vi "运维调试_五参数.vi"(11 "编号":string="001") -> ()   [LabVIEW 2016, in "斯坦道多参数.lvlib"]
uses:
  <vilib>/Utility/miscctls.llb/LVPointTypeDef.ctl
  <vilib>/Plasmionique/MB Master/MB_Master/MB_Master.lvclass
  <vilib>/Utility/config.llb/NI_LVConfig.lvlib
panel:
  out "权限等级":string
  in  "ORP校准":bool
  in  "ORP探头选择":u16(ring) items=["YL型", "MQ型", "NAQ型"]
  in  "ORP启用":bool
  in  "水样测量时间":dbl caption="水样测量时间:"
  in  "自动断线重连":bool=TRUE
  in  "打开modbus":bool
  out "选项卡控件":enum32{"选项卡 1", "选项卡 2"}(tab)
  in  "VISA资源名称":refnum<visa-resource-name> caption="串口"
  in  "IP":string="localhost" caption="IP:"
  in  "Port":u16=502 caption="Port:"
  in  "连接方式":u16(ring) items=["Modbus RTU", "Modbus TCP"]
  in  "藻密度校准":bool
  in  "密码锁":bool
  in  "藻密度探头选择":u16(ring) items=["YL型", "MQ型", "NAQ型"]
  in  "叶绿素a探头选择":u16(ring) items=["YL型", "MQ型", "NAQ型"]
  in  "浊度探头选择":u16(ring) items=["YL型", "MQ型", "NAQ型"]
  in  "电导率探头选择":u16(ring) items=["YL型", "MQ型", "NAQ型"]
  in  "DO探头选择":u16(ring) items=["YL型", "MQ型", "NAQ型"]
  in  "pH探头选择":u16(ring) items=["YL型", "MQ型", "NAQ型"]
  in  "设置页返回":bool
  in  "藻密度":bool
  in  "叶绿素a启用":bool
  in  "Temp":bool
  in  "Cond":bool
  in  "Turb":bool
  in  "DO":bool
  in  "pH":bool
  in  "周期设置":bool
  out "当前串口":string
  out "运行状态":u16(ring) items=["空闲", "水样测试", "标样核查"]
  in  "叶绿素a校准":bool
  in  "停止":bool
  in  "标样核查":bool
  in  "水样测试":bool
  in  "设置":bool
  in  "水温校准":bool
  in  "浊度校准":bool
  in  "溶解氧校准":bool
  in  "电导率校准":bool
  in  "pH校准":bool
  in  "探头校正返回":bool
  in  "探头校正":bool
  out "检测值":T1(array[cluster])
  # "请设置仪器连接方式"
  # "请选择要启用的参数"
  # "min"
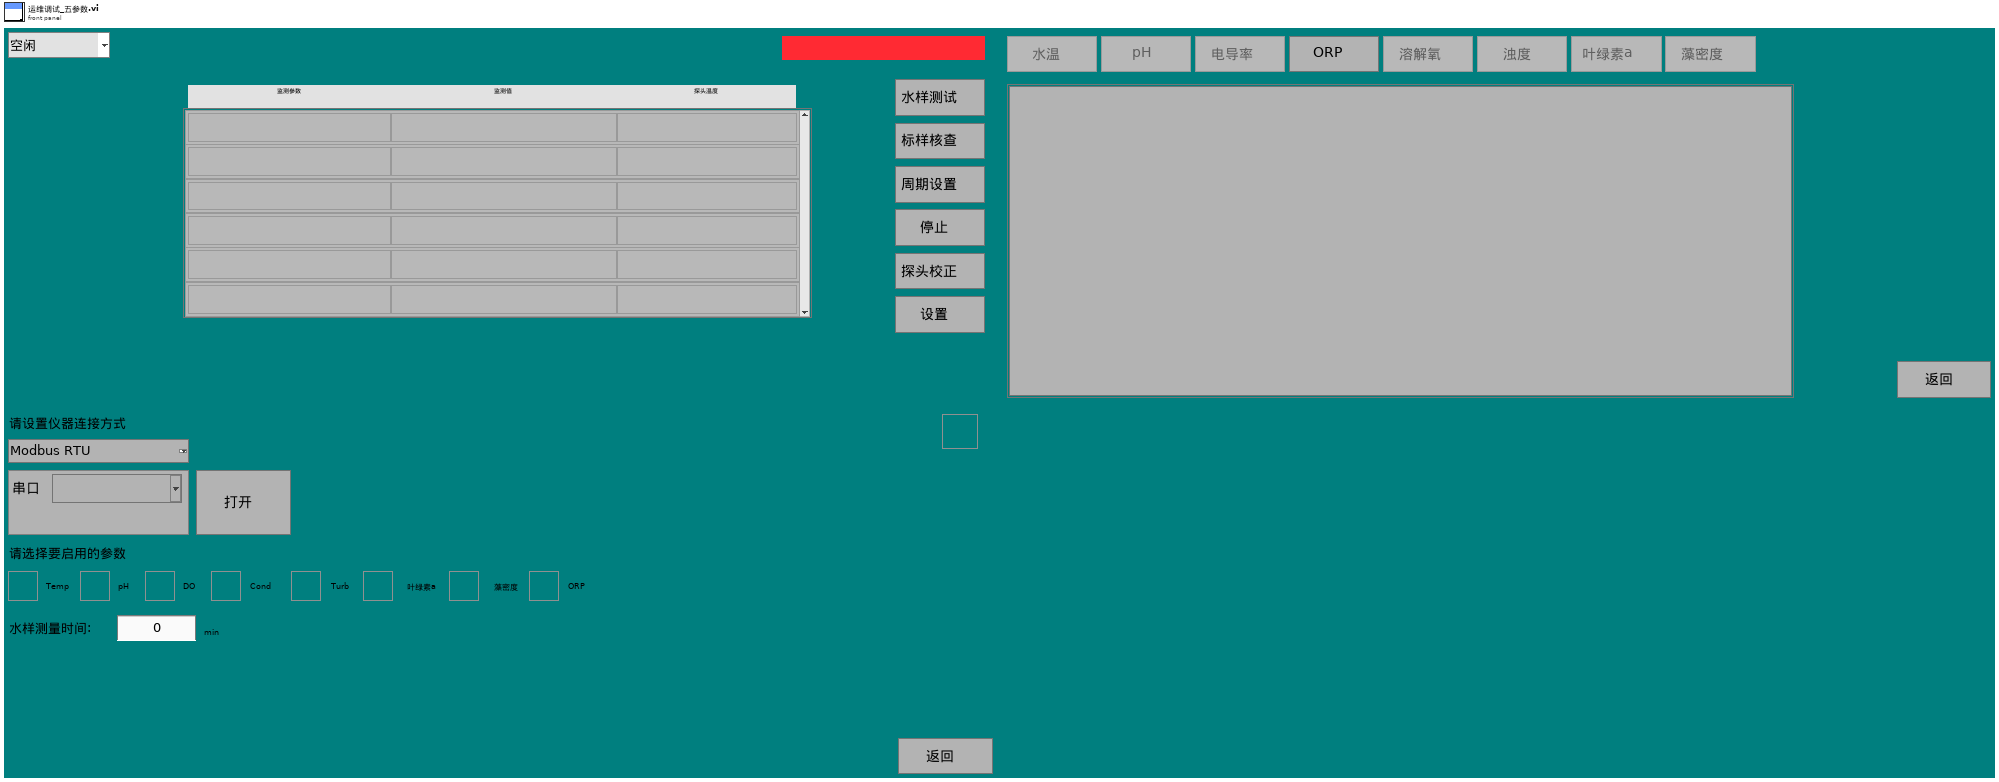
[diagram p1: front panel]
types:
  T1 = cluster{"监测参数1":string, "浓度1":string, "探头温度1":string}[]
  T2 = typedef "LVPointTypeDef.ctl" = cluster{"Horizontal":i16, "Vertical":i16}
  T3 = enum8{"Enabled", "Disabled", "Disabled and Grayed Out"}
  T4 = cluster{"pH探头选择":u16, "DO探头选择":u16, "电导率探头选择":u16, "浊度探头选择":u16, "叶绿素a探头选择":u16, "蓝绿藻探头选择":u16, "orp探头选择":u16}
  T5 = cluster{"温度测量值":sgl, "DO%":sgl, "DOmg/L":sgl, "温度偏移修正值":sgl}
  T6 = cluster{"周期设置类型":enum16{"定点启动", "间隔启动"}, "定时功能启用":bool, "定时间隔":u32, "24H周期设置":bool[]}
  T7 = enum32{"Bad", "Idle", "Run top level", "Running"}
  T8 = typedef "LVDateTimeRec.ctl" = cluster{"秒数的小数部分":dbl, "秒":i32, "分":i32, "时":i32, "日":i32, "月":i32, "年":i32, "天数（周）":i32, "天数（年）":i32, "DST":i32}
  T9 = typedef "NI_LVConfig.lvlib/Config Data RefNum.ctl" = refnum<k1>
  T10 = cluster{"pH校准VI引用句柄":refnum<vi>, "DO校准VI引用句柄":refnum<vi>, "COND校准VI引用句柄":refnum<vi>, "TURB校准VI引用句柄":refnum<vi>, "CHLA校准VI引用句柄":refnum<vi>, "BGA校准VI引用句柄":refnum<vi>, "ORP校准VI引用句柄":refnum<vi>}
  T11 = cluster{"数据保存间隔":dbl, "水温标样值":dbl, "pH标样值":dbl, "溶解氧标样值":dbl, "电导率标样值":dbl, "浊度标样值":dbl}
  T12 = cluster{"baud rate (bps)":u32, "stop bits":u16, "parity":u16, "flow control":u16, "timeout":u32, "retries":i32}
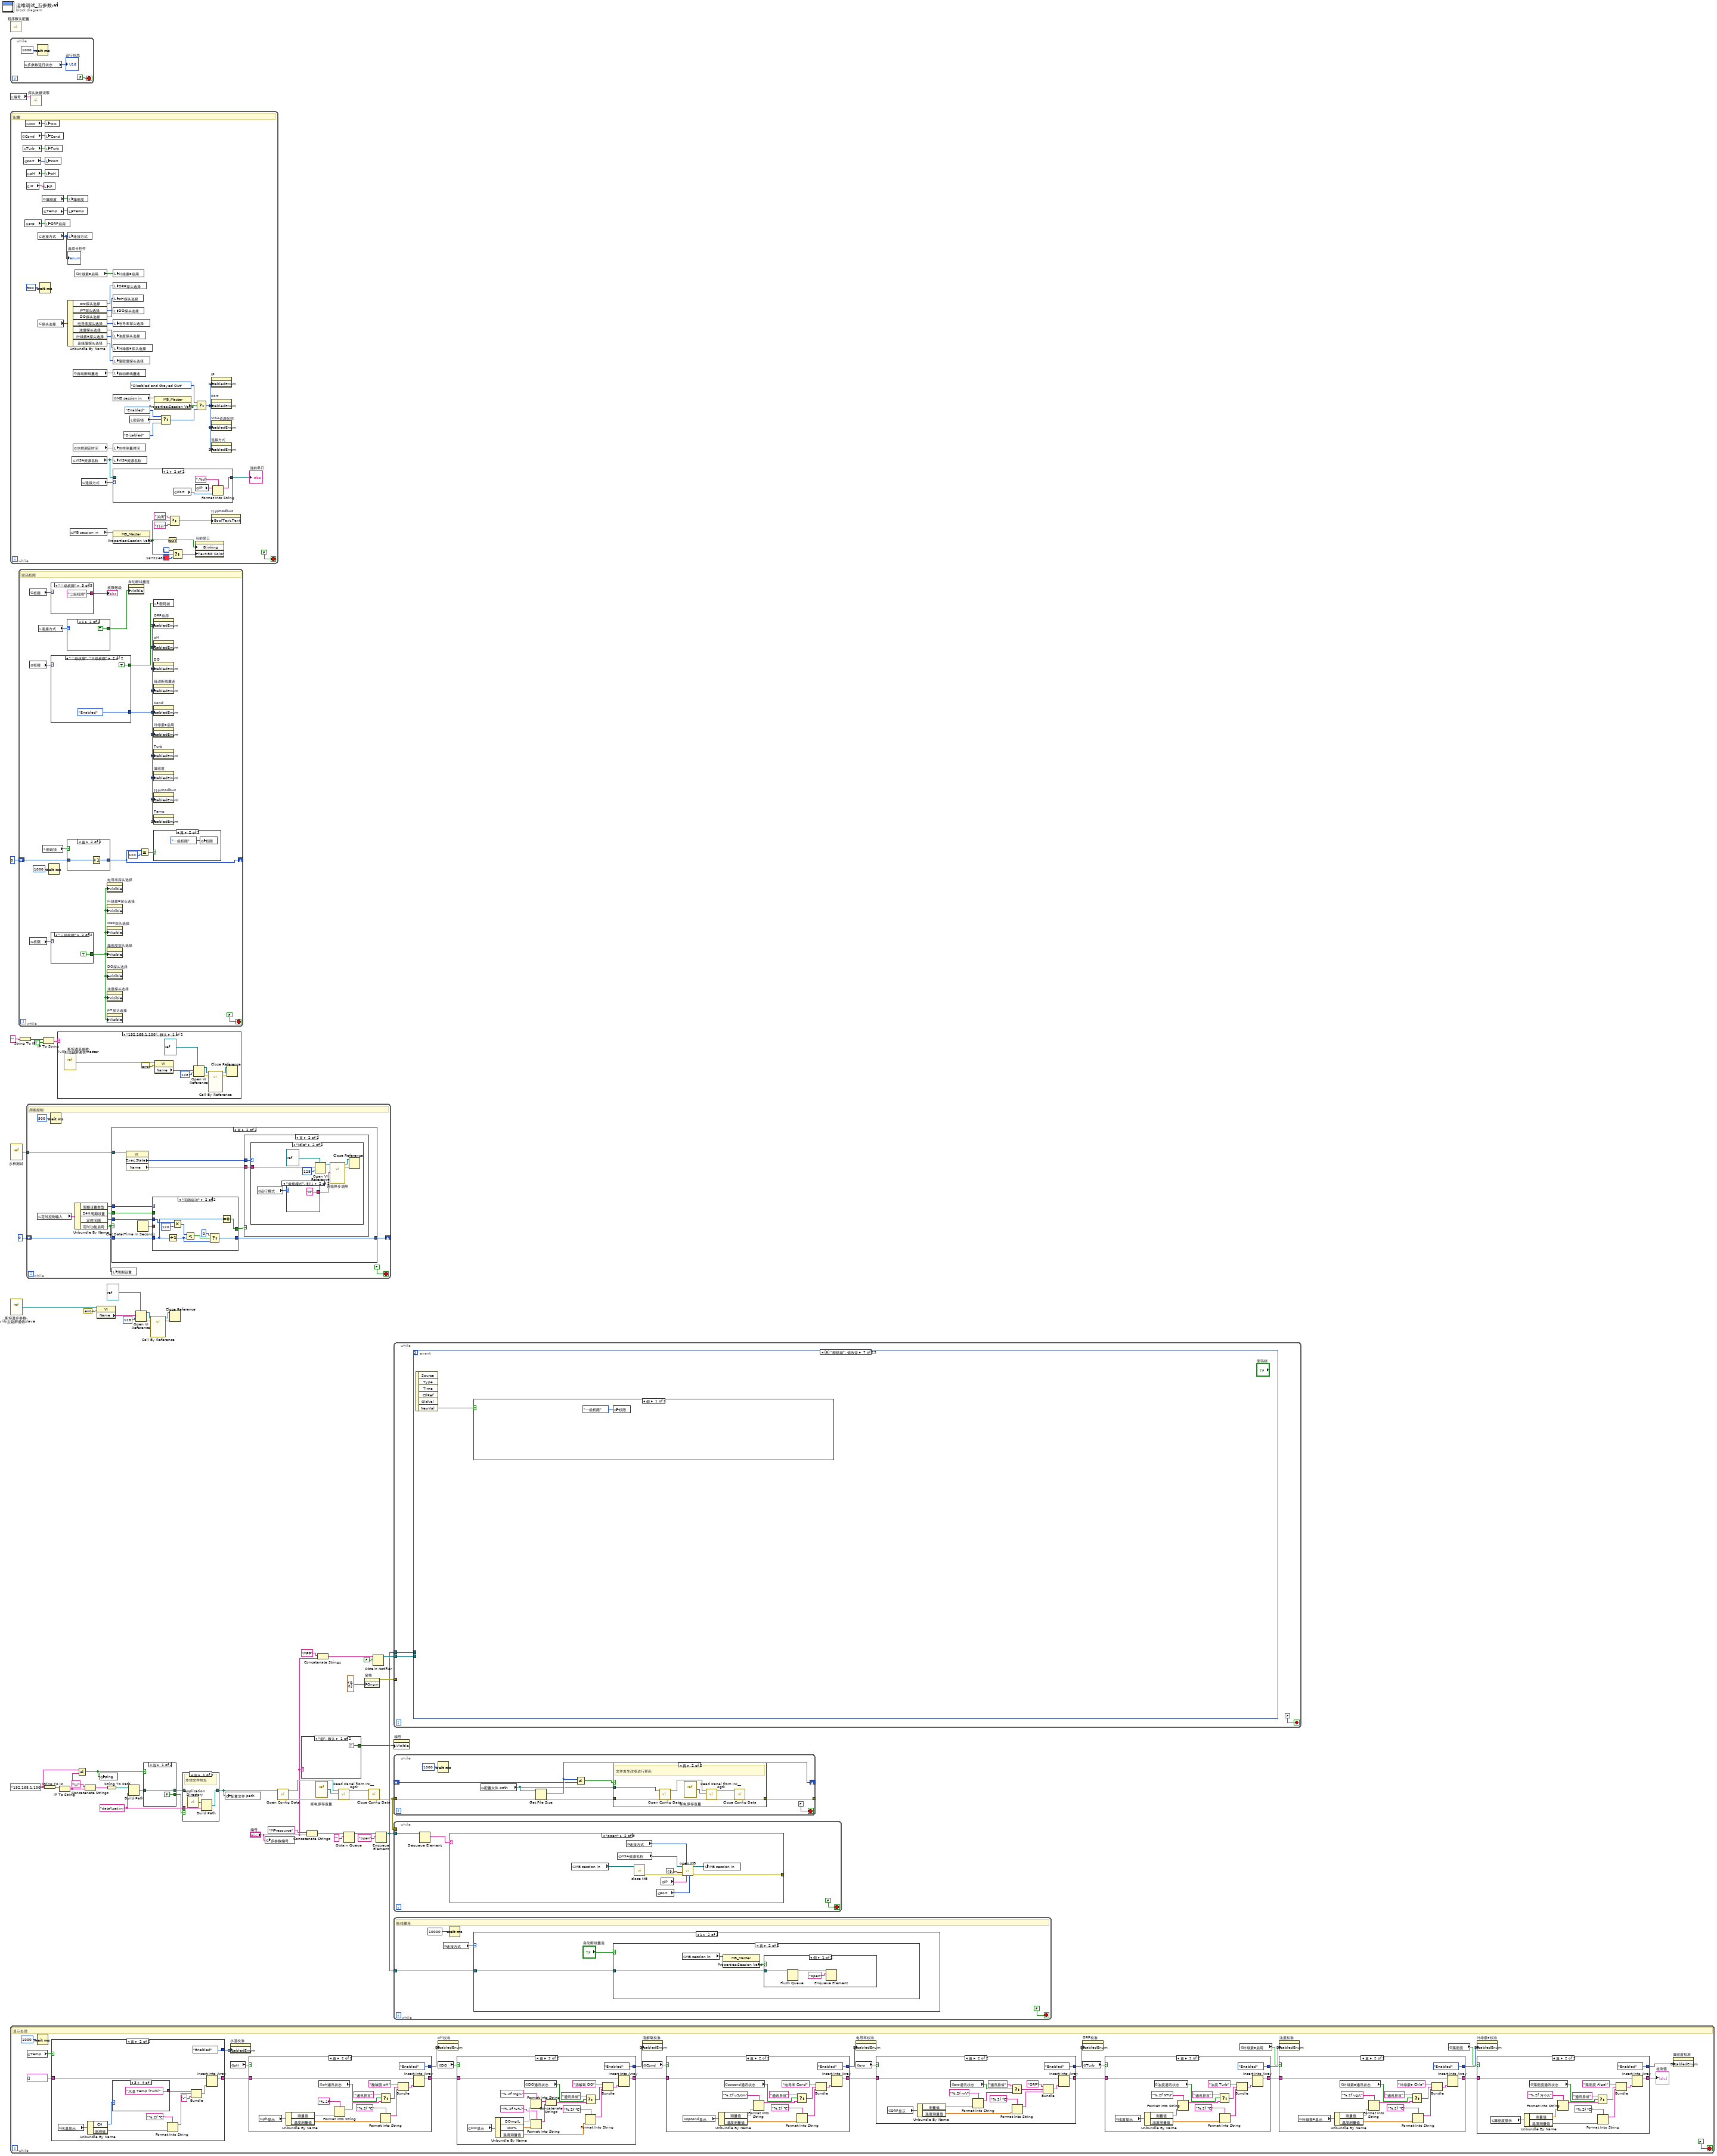
[diagram p0: block diagram]
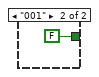
[diagram p2: hidden frame]
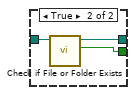
[diagram p4: hidden frame]
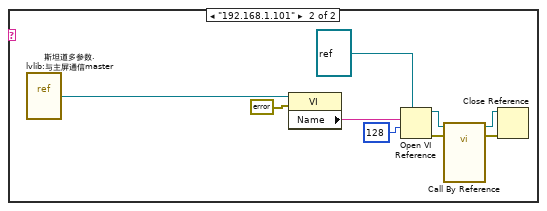
[diagram p6: hidden frame]
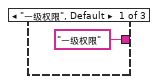
[diagram p13: hidden frame]
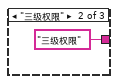
[diagram p14: hidden frame]
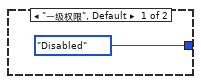
[diagram p15: hidden frame]
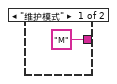
[diagram p20: hidden frame]
diagram:
  w16 = "data\\set.ini" ("名称或相对路径")
  w8 = "192.168.1.100" ("名称")
  n1 = call "程序默认配置.vi"() -> ()  [unwired: 11 in, 1 out]
  n2 = while {
    stop <- FALSE stop-if-true
    n3 = global read "多参数全局变量.vi" "多参数运行状态"() -> (→"运行状态":u16)
    n4 = Wait (ms)(milliseconds to wait=u32 1000 ("等待时间（毫秒）")) -> ()  [unwired: 1 out]
  }
  n5 = local read "编号"() -> (w3:string)
  n6 = while {
    stop <- FALSE stop-if-true
    # "配置"
    n7 = global read "断电保存变量.vi" "Cond"() -> (w91:bool)
    n8 = global read "断电保存变量.vi" "Turb"() -> (w90:bool)
    n9 = global read "断电保存变量.vi" "Port"() -> (w69:u16)
    n10 = global read "断电保存变量.vi" "orp"() -> (w54:bool)
    n11 = global read "断电保存变量.vi" "DO"() -> (w92:bool)
    n12 = global read "断电保存变量.vi" "pH"() -> (w93:bool)
    n13 = global read "断电保存变量.vi" "IP"() -> (w70:string)
    n14 = global read "断电保存变量.vi" "连接方式"() -> (w62:u16)
    "选项卡控件" <- w62
    n15 = global read "断电保存变量.vi" "探头选择"() -> (w80:T4)
    n16 = Wait (ms)(milliseconds to wait=u32 500 ("等待时间（毫秒）")) -> ()  [unwired: 1 out]
    n17 = global read "断电保存变量.vi" "藻密度"() -> (w88:bool)
    n18 = global read "断电保存变量.vi" "Temp"() -> (w94:bool)
    n19 = local write "IP"(w70) -> ()
    n20 = local write "DO"(w92) -> ()
    n21 = local write "Cond"(w91) -> ()
    n22 = local write "Turb"(w90) -> ()
    n23 = local write "Port"(w69) -> ()
    n24 = local write "pH"(w93) -> ()
    n25 = local write "ORP启用"(w54) -> ()
    n26 = local write "藻密度"(w88) -> ()
    n27 = local write "Temp"(w94) -> ()
    n28 = local write "连接方式"(w62) -> ()
    n29 = Unbundle By Name(w80) -> ("orp探头选择"=w53:u16, "pH探头选择"=w63:u16, "DO探头选择"=w79:u16, "电导率探头选择"=w78:u16, "浊度探头选择"=w77:u16, "叶绿素a探头选择"=w76:u16, "蓝绿藻探头选择"=w75:u16)
    n30 = global read "多参数全局变量.vi" "MB session in"() -> (w84:refnum<class "MB_Master.lvclass">)
    n31 = global read "断电保存变量.vi" "VISA资源名称"() -> (w66:refnum<visa-resource-name>)
    n32 = global read "断电保存变量.vi" "自动断线重连"() -> (w57:bool)
    n33 = global read "断电保存变量.vi" "水样测定时间"() -> (w56:dbl)
    n34 = global read "断电保存变量.vi" "叶绿素a启用"() -> (w89:bool)
    n35 = global read "断电保存变量.vi" "连接方式"() -> (w67:u16)
    n36 = local write "叶绿素a启用"(w89) -> ()
    n37 = local write "ORP探头选择"(w53) -> ()
    n38 = local write "pH探头选择"(w63) -> ()
    n39 = local write "DO探头选择"(w79) -> ()
    n40 = local write "电导率探头选择"(w78) -> ()
    n41 = local write "浊度探头选择"(w77) -> ()
    n42 = local write "叶绿素a探头选择"(w76) -> ()
    n43 = local write "藻密度探头选择"(w75) -> ()
    n44 = local write "自动断线重连"(w57) -> ()
    n45 = global read "多参数全局变量.vi" "MB session in"() -> (w87:refnum<class "MB_Master.lvclass">)
    n46 = local write "水样测量时间"(w56) -> ()
    n47 = local write "VISA资源名称"(w66) -> ()
    n48 = case shown="1" w67 {
      tunnel: w66 -> [w96 _]
      tunnel: [w96 w97] -> w65
      frame 0, Default {
      }
      frame 1 {
        n49 = global read "断电保存变量.vi" "Port"() -> (w98:u16)
        n50 = global read "断电保存变量.vi" "IP"() -> (w100:string)
        n51 = Format Into String(format string=":%d" ("格式字符串"), initial string=w100, w98) -> (resulting string=w97:string)  [unwired: 1 in, 1 out]
      }
    }
    "当前串口" <- w65
    n52 = property class="MB_Master"(reference=w84) -> ("Properties:Session Valid"=w61:bool)  [unwired: 1 in, 2 out]
    n53 = local read "密码锁"() -> (w74:bool)
    n54 = property class="MB_Master"(reference=w87) -> ("Properties:Session Valid"=w86:bool)  [unwired: 1 in, 2 out]
    n55 = Select(t=T3."Enabled" ("f"), s=w74, f=T3."Disabled") -> (s? t:f=w72:T3)
    n56 = Not(x=w61) -> (.not. x?=w64:bool)
    n57 = Select(t="关闭" ("布尔文本.文本"), s=w61, f="打开" ("布尔文本.文本")) -> (s? t:f=w81:string)
    n58 = Select(t=u32 16777216, s=w61, f=u32 16722483) -> (s? t:f=w58:u32)
    n59 = property on="当前串口" class="Str"("Blinking"=w64, "Text.BG Color"=w58) -> ()  [unwired: 2 in, 2 out]
    n60 = Select(t=T3."Disabled and Grayed Out" ("禁用"), s=w86, f=w72) -> (s? t:f=w68:T3)
    n61 = property on="IP" class="Str"("DisabledEnum"=w68) -> ()  [unwired: 2 in, 2 out]
    n62 = property on="Port" class="DigNum (严格)"("DisabledEnum"=w68) -> ()  [unwired: 2 in, 2 out]
    n63 = property on="VISA资源名称" class="VISAName"("DisabledEnum"=w68) -> ()  [unwired: 2 in, 2 out]
    n64 = property on="连接方式" class="Ring (严格)"("DisabledEnum"=w68) -> ()  [unwired: 2 in, 2 out]
    n65 = property on="打开modbus" class="Bool"("BoolText.Text"=w81) -> ()  [unwired: 2 in, 2 out]
  }
  n66 = vi-ref "水样测试.vi"() -> (w39:refnum<vi>)
  n67 = vi-ref "斯坦道多参数.lvlib:主副屏通信slave.vi"() -> (w21:refnum<vi>)
  n68 = while {
    stop <- FALSE stop-if-true
    # "显示处理"
    n69 = global read "断电保存变量.vi" "Temp"() -> (w125:bool)
    n70 = Wait (ms)(milliseconds to wait=u32 1000 ("等待时间（毫秒）")) -> ()  [unwired: 1 out]
    n71 = case shown="真" w125 {
      tunnel: [w252 w257] -> w122
      tunnel: T1 [] ("数组") -> [w252 w258]
      tunnel: [T3."Disabled and Grayed Out" ("禁用") T3."Enabled" ("禁用")] -> w109
      frame False {
      }
      frame True {
        n72 = global read "多参数全局变量.vi" "水温显示"() -> (w255:cluster{"CH":u16, "监测值":dbl, "温度偏移修正值":sgl})
        n73 = Unbundle By Name(w255) -> ("CH"=w254:u16, "监测值"=w253:dbl)
        n74 = case shown="3" w254 {
          tunnel: ["水温 Temp (pH)" ("监测参数1") "水温 Temp (Cond)" ("监测参数1") "水温 Temp (DO)" ("监测参数1") "水温 Temp (Turb)" ("监测参数1")] -> w262
          frame 0, Default {
          }
          frame 1 {
          }
          frame 2 {
          }
          frame 3 {
          }
        }
        n75 = Format Into String(format string="%.2f ℃" ("格式字符串"), w253) -> (resulting string=w261:string)  [unwired: 2 in, 1 out]
        n76 = Bundle("监测参数1"=w262, w261, "探头温度1"="-") -> (w259:cluster{"监测参数1":string, string, "探头温度1":string})  [unwired: 1 in]
        n77 = Insert Into Array(array=w258, new element=w259) -> (w257:T1)  [unwired: 1 in]
      }
    }
    n78 = property on="水温校准" class="Bool"("DisabledEnum"=w109) -> ()  [unwired: 2 in, 2 out]
    n79 = global read "断电保存变量.vi" "pH"() -> (w123:bool)
    n80 = case shown="真" w123 {
      tunnel: [w235 w242] -> w120
      tunnel: w122 -> [w235 w244]
      tunnel: [T3."Disabled and Grayed Out" ("禁用") T3."Enabled" ("禁用")] -> w114
      frame False {
      }
      frame True {
        n81 = global read "多参数全局变量.vi" "ph显示"() -> (w240:cluster{"温度测量值":sgl, "测量值":sgl, "温度偏移修正值":sgl})
        n82 = Unbundle By Name(w240) -> ("测量值"=w250:sgl, "温度测量值"=w248:sgl)
        n83 = global read "多参数全局变量.vi" "ph通讯状态"() -> (w238:bool)
        n84 = Format Into String(format string="%.2f" ("格式字符串"), w250) -> (resulting string=w237:string)  [unwired: 2 in, 1 out]
        n85 = Select(t="通讯异常" ("格式字符串"), s=w238, f=w237) -> (s? t:f=w236:string)
        n86 = Format Into String(format string="%.2f ℃" ("格式字符串"), w248) -> (resulting string=w246:string)  [unwired: 2 in, 1 out]
        n87 = Bundle("监测参数2"="酸碱度 pH", "格式字符串"=w236, w246) -> (w243:cluster{"监测参数2":string, "格式字符串":string, string})  [unwired: 1 in]
        n88 = Insert Into Array(array=w244, new element=w243) -> (w242:T1)  [unwired: 1 in]
      }
    }
    n89 = property on="pH校准" class="Bool"("DisabledEnum"=w114) -> ()  [unwired: 2 in, 2 out]
    n90 = global read "断电保存变量.vi" "DO"() -> (w121:bool)
    n91 = case shown="真" w121 {
      tunnel: [w214 w221] -> w117
      tunnel: w120 -> [w214 w222]
      tunnel: [T3."Disabled and Grayed Out" ("禁用") T3."Enabled" ("禁用")] -> w113
      frame False {
      }
      frame True {
        n92 = global read "多参数全局变量.vi" "DO显示"() -> (w219:T5)
        n93 = Unbundle By Name(w219) -> ("DOmg/L"=w230:sgl, "DO%"=w228:sgl, "温度测量值"=w232:sgl)
        n94 = global read "多参数全局变量.vi" "DO通讯状态"() -> (w217:bool)
        n95 = Format Into String(format string="%.2f mg/L" ("格式字符串"), w230) -> (resulting string=w227:string)  [unwired: 2 in, 1 out]
        n96 = Format Into String(format string="(%.2f %%)" ("格式字符串"), w228) -> (resulting string=w226:string)  [unwired: 2 in, 1 out]
        n97 = Concatenate Strings(w227, w226) -> (w216:string)
        n98 = Select(t="通讯异常" ("格式字符串"), s=w217, f=w216) -> (s? t:f=w215:string)
        n99 = Format Into String(format string="%.2f ℃" ("格式字符串"), w232) -> (resulting string=w224:string)  [unwired: 2 in, 1 out]
        n100 = Bundle("监测参数2"="溶解氧 DO", "格式字符串"=w215, w224) -> (w223:cluster{"监测参数2":string, "格式字符串":string, string})  [unwired: 1 in]
        n101 = Insert Into Array(array=w222, new element=w223) -> (w221:T1)  [unwired: 1 in]
      }
    }
    n102 = property on="溶解氧校准" class="Bool"("DisabledEnum"=w113) -> ()  [unwired: 2 in, 2 out]
    n103 = global read "断电保存变量.vi" "Cond"() -> (w119:bool)
    n104 = case shown="真" w119 {
      tunnel: w117 -> [w197 w208]
      tunnel: [w197 w198] -> w102
      tunnel: [T3."Disabled and Grayed Out" ("禁用") T3."Enabled" ("禁用")] -> w112
      frame False {
      }
      frame True {
        n105 = global read "多参数全局变量.vi" "spcond显示"() -> (w205:cluster{"温度测量值":sgl, "测量值":sgl, "温度偏移修正值":sgl})
        n106 = Unbundle By Name(w205) -> ("测量值"=w204:sgl, "温度测量值"=w203:sgl)
        n107 = global read "多参数全局变量.vi" "spcond通讯状态"() -> (w201:bool)
        n108 = Format Into String(format string="%.2f uS/cm" ("格式字符串"), w204) -> (resulting string=w200:string)  [unwired: 2 in, 1 out]
        n109 = Select(t="通讯异常" ("格式字符串"), s=w201, f=w200) -> (s? t:f=w199:string)
        n110 = Format Into String(format string="%.2f ℃" ("格式字符串"), w203) -> (resulting string=w209:string)  [unwired: 2 in, 1 out]
        n111 = Bundle("监测参数2"="电导率 Cond", "格式字符串"=w199, w209) -> (w207:cluster{"监测参数2":string, "格式字符串":string, string})  [unwired: 1 in]
        n112 = Insert Into Array(array=w208, new element=w207) -> (w198:T1)  [unwired: 1 in]
      }
    }
    n113 = property on="电导率校准" class="Bool"("DisabledEnum"=w112) -> ()  [unwired: 2 in, 2 out]
    n114 = global read "断电保存变量.vi" "orp"() -> (w104:bool)
    n115 = case shown="真" w104 {
      tunnel: w102 -> [w129 w140]
      tunnel: [w129 w138] -> w103
      tunnel: [T3."Disabled and Grayed Out" ("禁用") T3."Enabled" ("禁用")] -> w101
      frame False {
      }
      frame True {
        n116 = global read "多参数全局变量.vi" "ORP显示"() -> (w136:cluster{"温度测量值":sgl, "测量值":sgl, "温度偏移修正值":sgl})
        n117 = Unbundle By Name(w136) -> ("测量值"=w135:sgl, "温度测量值"=w134:sgl)
        n118 = global read "多参数全局变量.vi" "orp通讯状态"() -> (w132:bool)
        n119 = Format Into String(format string="%.2f mV" ("格式字符串"), w135) -> (resulting string=w131:string)  [unwired: 2 in, 1 out]
        n120 = Select(t="通讯异常" ("格式字符串"), s=w132, f=w131) -> (s? t:f=w130:string)
        n121 = Format Into String(format string="%.2f ℃" ("格式字符串"), w134) -> (resulting string=w141:string)  [unwired: 2 in, 1 out]
        n122 = Bundle("监测参数2"="ORP", "格式字符串"=w130, w141) -> (w139:cluster{"监测参数2":string, "格式字符串":string, string})  [unwired: 1 in]
        n123 = Insert Into Array(array=w140, new element=w139) -> (w138:T1)  [unwired: 1 in]
      }
    }
    n124 = property on="ORP校准" class="Bool"("DisabledEnum"=w101) -> ()  [unwired: 2 in, 2 out]
    n125 = global read "断电保存变量.vi" "Turb"() -> (w118:bool)
    n126 = case shown="真" w118 {
      tunnel: w103 -> [w180 w191]
      tunnel: [w180 w189] -> w116
      tunnel: [T3."Disabled and Grayed Out" ("禁用") T3."Enabled" ("禁用")] -> w111
      frame False {
      }
      frame True {
        n127 = global read "多参数全局变量.vi" "浊度显示"() -> (w187:cluster{"温度测量值":sgl, "测量值":sgl, "温度偏移修正值":sgl})
        n128 = Unbundle By Name(w187) -> ("测量值"=w186:sgl, "温度测量值"=w185:sgl)
        n129 = global read "多参数全局变量.vi" "浊度通讯状态"() -> (w183:bool)
        n130 = Format Into String(format string="%.2f NTU" ("格式字符串"), w186) -> (resulting string=w182:string)  [unwired: 2 in, 1 out]
        n131 = Select(t="通讯异常" ("格式字符串"), s=w183, f=w182) -> (s? t:f=w181:string)
        n132 = Format Into String(format string="%.2f ℃" ("格式字符串"), w185) -> (resulting string=w193:string)  [unwired: 2 in, 1 out]
        n133 = Bundle("监测参数2"="浊度 Turb", "格式字符串"=w181, w193) -> (w190:cluster{"监测参数2":string, "格式字符串":string, string})  [unwired: 1 in]
        n134 = Insert Into Array(array=w191, new element=w190) -> (w189:T1)  [unwired: 1 in]
      }
    }
    n135 = global read "断电保存变量.vi" "叶绿素a启用"() -> (w115:bool)
    n136 = property on="浊度校准" class="Bool"("DisabledEnum"=w111) -> ()  [unwired: 2 in, 2 out]
    n137 = case shown="真" w115 {
      tunnel: w116 -> [w163 w174]
      tunnel: [w163 w172] -> w106
      tunnel: [T3."Disabled and Grayed Out" ("禁用") T3."Enabled" ("禁用")] -> w110
      frame False {
      }
      frame True {
        n138 = global read "多参数全局变量.vi" "叶绿素a显示"() -> (w168:cluster{"温度测量值":sgl, "测量值":sgl, "温度偏移修正值":sgl})
        n139 = Unbundle By Name(w168) -> ("测量值"=w171:sgl, "温度测量值"=w170:sgl)
        n140 = global read "多参数全局变量.vi" "叶绿素a通讯状态"() -> (w166:bool)
        n141 = Format Into String(format string="%.2f ug/L" ("格式字符串"), w171) -> (resulting string=w165:string)  [unwired: 2 in, 1 out]
        n142 = Select(t="通讯异常" ("格式字符串"), s=w166, f=w165) -> (s? t:f=w164:string)
        n143 = Format Into String(format string="%.2f ℃" ("格式字符串"), w170) -> (resulting string=w176:string)  [unwired: 2 in, 1 out]
        n144 = Bundle("监测参数2"="叶绿素a Chla", "格式字符串"=w164, w176) -> (w173:cluster{"监测参数2":string, "格式字符串":string, string})  [unwired: 1 in]
        n145 = Insert Into Array(array=w174, new element=w173) -> (w172:T1)  [unwired: 1 in]
      }
    }
    n146 = global read "断电保存变量.vi" "藻密度"() -> (w107:bool)
    n147 = property on="叶绿素a校准" class="Bool"("DisabledEnum"=w110) -> ()  [unwired: 2 in, 2 out]
    n148 = case shown="真" w107 {
      tunnel: w106 -> [w146 w157]
      tunnel: [w146 w155] -> w105
      tunnel: [T3."Disabled and Grayed Out" ("禁用") T3."Enabled" ("禁用")] -> w108
      frame False {
      }
      frame True {
        n149 = global read "多参数全局变量.vi" "藻密度显示"() -> (w151:cluster{"温度测量值":sgl, "测量值":sgl, "温度偏移修正值":sgl})
        n150 = Unbundle By Name(w151) -> ("测量值"=w154:sgl, "温度测量值"=w153:sgl)
        n151 = global read "多参数全局变量.vi" "藻密度通讯状态"() -> (w149:bool)
        n152 = Format Into String(format string="%.2f 万个/L" ("格式字符串"), w154) -> (resulting string=w148:string)  [unwired: 2 in, 1 out]
        n153 = Select(t="通讯异常" ("格式字符串"), s=w149, f=w148) -> (s? t:f=w147:string)
        n154 = Format Into String(format string="%.2f ℃" ("格式字符串"), w153) -> (resulting string=w159:string)  [unwired: 2 in, 1 out]
        n155 = Bundle("监测参数2"="藻密度 Algal", "格式字符串"=w147, w159) -> (w156:cluster{"监测参数2":string, "格式字符串":string, string})  [unwired: 1 in]
        n156 = Insert Into Array(array=w157, new element=w156) -> (w155:T1)  [unwired: 1 in]
      }
    }
    "检测值" <- w105
    n157 = property on="藻密度校准" class="Bool"("DisabledEnum"=w108) -> ()  [unwired: 2 in, 2 out]
  }
  n158 = while {
    shift-right: [w279] -> _
    shift-left: u32 0 ("等待时间（毫秒）") -> [w280]
    stop <- FALSE stop-if-true
    # "密码权限"
    n159 = global read "多参数全局变量.vi" "权限"() -> (w271:enum16{"一级权限", "二级权限", "三级权限"})
    n160 = global read "多参数全局变量.vi" "权限"() -> (w269:enum16{"一级权限", "二级权限", "三级权限"})
    n161 = global read "多参数全局变量.vi" "权限"() -> (w270:enum16{"一级权限", "二级权限", "三级权限"})
    n162 = local read "连接方式"() -> (w276:u16)
    n163 = local read "密码锁"() -> (w281:bool)
    n164 = Wait (ms)(milliseconds to wait=u32 1000 ("等待时间（毫秒）")) -> ()  [unwired: 1 out]
    n165 = case shown="\"二级权限\"" w271 {
      tunnel: ["一级权限" ("权限等级") "三级权限" ("权限等级") "二级权限" ("权限等级")] -> w272
      frame "一级权限", Default {
      }
      frame "三级权限" {
      }
      frame "二级权限" {
      }
    }
    "权限等级" <- w272
    n166 = case shown="\"二级权限\", \"三级权限\"" w269 {
      tunnel: [T3."Disabled" ("禁用") T3."Enabled" ("禁用")] -> w274
      tunnel: [_ TRUE ("可见")] -> w268
      frame "一级权限", Default {
      }
      frame "二级权限", "三级权限" {
      }
    }
    n167 = case shown="\"三级权限\"" w270 {
      tunnel: [_ TRUE ("可见")] -> w273
      frame "一级权限", Default {
      }
      frame "三级权限" {
      }
    }
    n168 = case shown="1" w276 {
      tunnel: [_ TRUE ("可见")] -> w275
      frame 0, Default {
      }
      frame 1 {
      }
    }
    n169 = case shown="真" w281 {
      tunnel: w280 -> [_ w287]
      tunnel: [_ w286] -> w279
      frame False {
      }
      frame True {
        n170 = Increment(x=w287) -> (x+1=w286:u32)
      }
    }
    n171 = property on="电导率探头选择" class="Ring (严格)"("Visible"=w273) -> ()  [unwired: 2 in, 2 out]
    n172 = property on="叶绿素a探头选择" class="Ring (严格)"("Visible"=w273) -> ()  [unwired: 2 in, 2 out]
    n173 = property on="ORP探头选择" class="Ring (严格)"("Visible"=w273) -> ()  [unwired: 2 in, 2 out]
    n174 = property on="藻密度探头选择" class="Ring (严格)"("Visible"=w273) -> ()  [unwired: 2 in, 2 out]
    n175 = property on="DO探头选择" class="Ring (严格)"("Visible"=w273) -> ()  [unwired: 2 in, 2 out]
    n176 = property on="浊度探头选择" class="Ring (严格)"("Visible"=w273) -> ()  [unwired: 2 in, 2 out]
    n177 = property on="pH探头选择" class="Ring (严格)"("Visible"=w273) -> ()  [unwired: 2 in, 2 out]
    n178 = property on="自动断线重连" class="Bool (严格)"("Visible"=w275) -> ()  [unwired: 2 in, 2 out]
    n179 = Greater Or Equal?(x=w279, y=u32 120) -> (x >= y?=w277:bool)
    n180 = local write "密码锁"(w268) -> ()
    n181 = property on="ORP启用" class="Bool (严格)"("DisabledEnum"=w274) -> ()  [unwired: 2 in, 2 out]
    n182 = property on="pH" class="Bool (严格)"("DisabledEnum"=w274) -> ()  [unwired: 2 in, 2 out]
    n183 = property on="DO" class="Bool (严格)"("DisabledEnum"=w274) -> ()  [unwired: 2 in, 2 out]
    n184 = property on="自动断线重连" class="Bool (严格)"("DisabledEnum"=w274) -> ()  [unwired: 2 in, 2 out]
    n185 = property on="Cond" class="Bool (严格)"("DisabledEnum"=w274) -> ()  [unwired: 2 in, 2 out]
    n186 = property on="叶绿素a启用" class="Bool (严格)"("DisabledEnum"=w274) -> ()  [unwired: 2 in, 2 out]
    n187 = property on="Turb" class="Bool (严格)"("DisabledEnum"=w274) -> ()  [unwired: 2 in, 2 out]
    n188 = property on="藻密度" class="Bool (严格)"("DisabledEnum"=w274) -> ()  [unwired: 2 in, 2 out]
    n189 = property on="打开modbus" class="Bool"("DisabledEnum"=w274) -> ()  [unwired: 2 in, 2 out]
    n190 = property on="Temp" class="Bool (严格)"("DisabledEnum"=w274) -> ()  [unwired: 2 in, 2 out]
    n191 = case shown="真" w277 {
      frame False {
      }
      frame True {
        n192 = global write "多参数全局变量.vi" "权限"(enum16{"一级权限", "二级权限", "三级权限"}."一级权限" ("权限")) -> ()
      }
    }
  }
  n193 = String To IP(1:"" ("名称")) -> (0:w20:u32)
  n194 = while {
    tunnel: w39 -> [w297]
    shift-right: [w296] -> _
    shift-left: u32 0 ("等待时间（毫秒）") -> [w298]
    stop <- FALSE stop-if-true
    # "周期控制"
    n195 = global read "断电保存变量.vi" "定时控制输入"() -> (w300:T6)
    n196 = Wait (ms)(milliseconds to wait=u32 500 ("等待时间（毫秒）")) -> ()  [unwired: 1 out]
    n197 = Unbundle By Name(w300) -> ("周期设置类型"=w302:enum16{"定点启动", "间隔启动"}, "24H周期设置"=w301:bool[], "定时间隔"=w299:u32, "定时功能启用"=w295:bool)
    n198 = case shown="真" w295 {
      tunnel: w302 -> [_ w313]
      tunnel: w301 -> [_ w312]
      tunnel: w299 -> [_ w310]
      tunnel: w298 -> [_ w306]
      tunnel: w297 -> [_ w309]
      tunnel: [_ w305] -> w296
      frame False {
      }
      frame True {
        n199 = property class="VI"(reference=w309) -> ("Exec.State"=w307:T7, "Name"=w308:string)  [unwired: 1 in, 2 out]
        n200 = Get Date/Time In Seconds() -> (seconds since 1Jan1904=w314:timestamp)
        n201 = case shown="\"间隔启动\"" w313 {
          tunnel: w314 -> [w336 _]
          tunnel: w312 -> [w333 _]
          tunnel: [w327 w344] -> w311
          tunnel: w310 -> [_ w343]
          tunnel: w306 -> [_ w345]
          tunnel: [_ w339] -> w305
          frame "定点启动", Default {
            n202 = Seconds To Date/Time(time stamp (now)=w336) -> (date time rec=w335:T8)  [unwired: 1 in]
            n203 = Unbundle By Name(w335) -> ("时"=w334:i32, "分"=w332:i32, "秒"=w331:i32)
            n204 = Index Array(array=w333, index=w334) -> (element=w330:bool)
            n205 = Equal To 0?(x=w332) -> (x = 0?=w329:bool)
            n206 = Equal To 0?(x=w331) -> (x = 0?=w328:bool)
            n207 = Compound Arithmetic op=AND ("复合运算")(w330, w329, w328) -> (w327:bool)
          }
          frame "间隔启动" {
            n208 = Increment(x=w345) -> (x+1=w338:u32)
            n209 = Multiply(x=w343, y=u32 120) -> (x*y=w337:u32)
            n210 = Less?(x=w337, y=w338) -> (x < y?=w341:bool)
            n211 = Select(t=u32 0 ("y"), s=w341, f=w338) -> (s? t:f=w339:u32)
            n212 = Equal To 0?(x=w345) -> (x = 0?=w344:bool)
          }
        }
        n213 = case shown="真" w311 {
          tunnel: w307 -> [_ w316]
          tunnel: w308 -> [_ w315]
          frame False {
          }
          frame True {
            n214 = case shown="\"Idle\"" w316 {
              tunnel: w315 -> [_ w321]
              frame "Bad", Default {
              }
              frame "Idle" {
                n215 = global read "多参数全局变量.vi" "运行模式"() -> (w319:enum16{"维护模式", "常规模式", "应急模式", "质控模式"})
                n216 = case shown="\"常规模式\", 默认" w319 {
                  tunnel: ["M" ("数据标记表") "N" ("数据标记表")] -> w318
                  frame "维护模式" {
                  }
                  frame "常规模式", Default {
                  }
                }
                n217 = Open VI Reference(type specifier VI Refnum (for type only)=refnum<vi> refnum, vi path=w321, options=128 ("选项")) -> (vi reference=w322:refnum<vi>)  [unwired: 3 in, 1 out]
                n218 = call-by-ref "开始异步调用"(reference=w322, "数据标记表"=w318) -> (reference out=w323:refnum<vi>, error out=w324:errorcluster)  [unwired: 12 in]
                n219 = Close Reference(reference=w323, error in (no error)=w324) -> ()  [unwired: 1 out]
              }
            }
          }
        }
      }
    }
    n220 = local write "周期设置"(w295) -> ()
  }
  n221 = call "探头数据读取.vi"("编号"=w3) -> ()  [unwired: 11 in]
  n222 = IP To String(1:TRUE ("句点符号？(F)"), 2:w20) -> (0:w17:string)
  n223 = String To IP(1:w8) -> (0:w15:u32)
  n224 = case shown="\"192.168.1.100\", 默认" w17 {
    frame "192.168.1.100", Default {
      n225 = vi-ref "斯坦道多参数.lvlib:与副屏通信master.vi"() -> (w346:refnum<vi>)
      n226 = property class="VI"(reference=w346, error in=errorcluster {"status"=FALSE, "code"=0, "source"=""} ("错误输出")) -> ("Name"=w347:string)  [unwired: 2 out]
      n227 = Open VI Reference(type specifier VI Refnum (for type only)=refnum<vi> refnum, vi path=w347, options=128 ("选项")) -> (vi reference=w349:refnum<vi>, error out=w351:errorcluster)  [unwired: 3 in]
      n228 = call-by-ref "?"(reference=w349, error in=w351) -> (reference out=w353:refnum<vi>, error out=w352:errorcluster)  [unwired: 12 in]
      n229 = Close Reference(reference=w353, error in (no error)=w352) -> ()  [unwired: 1 out]
    }
    frame "192.168.1.101" {
      n230 = vi-ref "斯坦道多参数.lvlib:与主屏通信master.vi"() -> (w355:refnum<vi>)
      n231 = property class="VI"(reference=w355, error in=errorcluster {"status"=FALSE, "code"=0, "source"=""} ("错误输出")) -> ("Name"=w356:string)  [unwired: 2 out]
      n232 = Open VI Reference(type specifier VI Refnum (for type only)=refnum<vi> refnum, vi path=w356, options=128 ("选项")) -> (vi reference=w358:refnum<vi>, error out=w360:errorcluster)  [unwired: 3 in]
      n233 = call-by-ref "?"(reference=w358, error in=w360) -> (reference out=w362:refnum<vi>, error out=w361:errorcluster)  [unwired: 12 in]
      n234 = Close Reference(reference=w362, error in (no error)=w361) -> ()  [unwired: 1 out]
    }
  }
  n235 = IP To String(2:w15) -> (0:w12:string)  [unwired: 1 in]
  n236 = Not Equal?(x=w8, y=w12) -> (x != y?=w6:bool)
  n237 = Concatenate Strings("\\\\" ("字符串"), w12) -> (w13:string)
  n238 = property class="VI"(reference=w21, error in=errorcluster {"status"=FALSE, "code"=0, "source"=""} ("错误输出")) -> ("Name"=w22:string)  [unwired: 2 out]
  n239 = global write "多参数全局变量.vi" "ping"(w6) -> ()
  n240 = String To Path(string=w13) -> (path=w7:path)
  n241 = Build Path(base path=w7, name or relative path=w16) -> (appended path=w11:path)
  n242 = Open VI Reference(type specifier VI Refnum (for type only)=refnum<vi> refnum, vi path=w22, options=128 ("选项")) -> (vi reference=w24:refnum<vi>, error out=w26:errorcluster)  [unwired: 3 in]
  n243 = case shown="假" w6 {
    tunnel: w11 -> [w364 w368]
    tunnel: [w364 w367] -> w10
    tunnel: [FALSE w366] -> w9
    frame False {
    }
    frame True {
      n244 = call <vilib>:"Check if File or Folder Exists.vi"("path"=w368) -> ("file or folder exists?"=w366:bool, "dup path"=w367:path)  [unwired: 8 in, 1 out]
    }
  }
  n245 = call-by-ref "?"(reference=w24, error in=w26) -> (reference out=w28:refnum<vi>, error out=w27:errorcluster)  [unwired: 12 in]
  n246 = Close Reference(reference=w28, error in (no error)=w27) -> ()  [unwired: 1 out]
  n247 = case shown="假" w9 {
    tunnel: w10 -> [_ w372]
    tunnel: [w370 w372] -> w5
    tunnel: w16 -> [w369 _]
    frame False {
      # "本地文件地址"
      n248 = call <vilib>:"Application Directory.vi"() -> ("Application Directory"=w371:path)
      n249 = Build Path(base path=w371, name or relative path=w369) -> (appended path=w370:path)
    }
    frame True {
      # "网络共享地址"
    }
  }
  n250 = global write "多参数全局变量.vi" "配置文件 path"(w5) -> ()
  n251 = global write "多参数全局变量.vi" "多参数编号"("编号") -> ()
  n252 = call <vilib>:"Open Config Data.vi"("configuration file path"=w5) -> ("error out"=w33:errorcluster, "refnum"=w34:T9)  [unwired: 8 in, 1 out]
  n253 = case shown="\"假\", 默认" "编号" {
    tunnel: [TRUE ("可见") FALSE ("可见")] -> w1
    frame "假", Default {
    }
    frame "001" {
    }
  }
  n254 = Concatenate Strings("MPresource" ("名称（未命名）"), "编号") -> (w41:string)
  n255 = vi-ref "断电保存变量.vi"() -> (w30:refnum<vi>)
  n256 = Concatenate Strings("MPP" ("名称（未命名）"), "编号") -> (w42:string)
  n257 = call <userlib>:"Read Panel from INI__ogtk.vi"("error in (no error)"=w33, "VI ref"=w30, "refnum"=w34) -> ("error out"=w31:errorcluster, "refnum out"=w32:T9)  [unwired: 7 in]
  n258 = Obtain Queue(name (unnamed)=w41, element data type="" ("名称（未命名）")) -> (queue out=w37:refnum<queue>)  [unwired: 3 in, 2 out]
  n259 = property on="窗格" class="Pane"("Origin"=T2 {"Horizontal"=0, "Vertical"=0} ("原点")) -> (error out=w49:errorcluster)  [unwired: 2 in, 1 out]
  n260 = call <vilib>:"Close Config Data.vi"("error in (no error)"=w31, "refnum"=w32) -> ("error out"=w4:errorcluster)  [unwired: 8 in, 1 out]
  n261 = Obtain Notifier(name (unnamed)=w42, notification data type=FALSE) -> (notifier out=w45:refnum<notifier>)  [unwired: 2 in, 2 out]
  n262 = Enqueue Element(queue=w37, element="open" ("元素")) -> (queue out=w36:refnum<queue>)  [unwired: 2 in, 2 out]
  n263 = while {
    tunnel: w49 -> [_]
    tunnel: w45 -> [w376]
    tunnel: w36 -> [w375]
    stop <- FALSE stop-if-true
    n264 = event shown="[6] \"密码锁\": 值改变" {
      selector: _ -> [_ _ _ _ _ _ _ _ _ _ _ _ _ _ _ _ _ _ _ _ _ _ _]
      dyn-events: _ -> [_ _ _ _ _ _ _ _ _ _ _ _ _ _ _ _ _ _ _ _ _ _ _]
      timeout: _ -> [_ _ _ _ _ _ _ _ _ _ _ _ _ _ _ _ _ _ _ _ _ _ _]
      tunnel: w376 -> [_ _ _ _ _ _ _ _ _ _ w481 _ _ _ _ _ _ _ _ _ _ _ _]
      tunnel: w375 -> [_ _ _ _ _ _ _ _ _ _ _ _ _ w498 _ _ _ _ _ _ _ _ _]
      event Timeout {
        n265 = event-data() -> ()  [unwired: 1 in, 3 out]
      }
      event "水样测量时间": Mouse Down {
        n266 = event-data() -> ("CtlRef"=w378:refnum<vi>)  [unwired: 1 in, 5 out]
        n267 = property class="DigNum (严格)"(reference=w378) -> (reference out=w381:refnum<vi>, "Value"=w380:dbl)  [unwired: 1 in, 1 out]
        n268 = call "数字键盘.vi"("OldNumber"=w380) -> ("NewNumber"=w379:dbl)  [unwired: 1 in]
        n269 = property class="DigNum (严格)"(reference=w381, "Val(Sgnl)"=w379) -> ()  [unwired: 1 in, 2 out]
      }
      event "pH探头选择", "DO探头选择", "电导率探头选择", "浊度探头选择", "叶绿素a探头选择", "藻密度探头选择", "ORP探头选择": Value Change {
        n270 = event-data() -> ("CtlRef"=w382:refnum<vi>, "NewVal"=w383:u16)  [unwired: 1 in, 4 out]
        n271 = Two Button Dialog(message="请再次确认修改的型号是否与实际匹配，否则将导致通讯异常，并且此操作将终止所有正在校准的参数！" ("消息")) -> (T button?=w384:bool)  [unwired: 2 in]
        n272 = case shown="真" w384 {
          tunnel: w383 -> [_ w387]
          tunnel: w382 -> [_ w386]
          frame False {
          }
          frame True {
            n273 = flat-sequence {
              tunnel: w387 -> [w388]
              tunnel: w386 -> [w392]
              frame #0 {
                n274 = property class="Ring (严格)"(reference=w392) -> ("Label.Text"=w391:string)  [unwired: 1 in, 2 out]
                n275 = global read "断电保存变量.vi" "探头选择"() -> (w390:T4)
                n276 = global read "多参数全局变量.vi" "校准VI引用句柄"() -> (w393:T10)
                n277 = case shown="\"ORP探头选择\"" w391 {
                  tunnel: w390 -> [w395 w398 w401 w404 w407 w410 w413 w416]
                  tunnel: [w395 w397 w400 w403 w406 w409 w412 w415] -> w389
                  tunnel: w388 -> [_ w396 w399 w402 w405 w408 w411 w414]
                  frame Default {
                  }
                  frame "pH探头选择" {
                    n278 = Bundle By Name(cluster=w398, "pH探头选择"=w396) -> (w397:T4)
                  }
                  frame "电导率探头选择" {
                    n279 = Bundle By Name(cluster=w401, "电导率探头选择"=w399) -> (w400:T4)
                  }
                  frame "DO探头选择" {
                    n280 = Bundle By Name(cluster=w404, "DO探头选择"=w402) -> (w403:T4)
                  }
                  frame "浊度探头选择" {
                    n281 = Bundle By Name(cluster=w407, "浊度探头选择"=w405) -> (w406:T4)
                  }
                  frame "叶绿素a探头选择" {
                    n282 = Bundle By Name(cluster=w410, "叶绿素a探头选择"=w408) -> (w409:T4)
                  }
                  frame "蓝绿藻探头选择" {
                    n283 = Bundle By Name(cluster=w413, "蓝绿藻探头选择"=w411) -> (w412:T4)
                  }
                  frame "ORP探头选择" {
                    n284 = Bundle By Name(cluster=w416, "蓝绿藻探头选择"=w414) -> (w415:T4)
                  }
                }
                n285 = Cluster To Array(cluster=w393) -> (array=w394:refnum<vi>[])
                n286 = for {
                  tunnel: w394 -> [w418] mode=indexing
                  tunnel: [w417] -> _ mode=indexing
                  n287 = invoke class="VI" method="Abort VI"(reference=w418) -> (error out=w417:errorcluster)  [unwired: 2 in, 2 out]
                }
                n288 = global write "断电保存变量.vi" "探头选择"(w389) -> ()
              }
              frame #1 {
                n289 = call "配置文件保存.vi"() -> ()  [unwired: 12 in]
              }
            }
          }
        }
      }
      event "VISA资源名称", "pH", "DO", "Turb", "Cond", "Temp", "叶绿素a启用", "打开modbus", "藻密度", "连接方式", "自动断线重连", "ORP启用": Mouse Down {
        n290 = event-data() -> ()  [unwired: 1 in, 6 out]
        n291 = local read "密码锁"() -> (w419:bool)
        n292 = case shown="假" w419 {
          frame False {
            n293 = One Button Dialog(message="当前操作权限不足,请提升权限!!!" ("消息")) -> ()  [unwired: 1 in, 1 out]
          }
          frame True {
          }
        }
      }
      event "IP": Mouse Down {
        n294 = event-data() -> ("CtlRef"=w422:refnum<vi>)  [unwired: 1 in, 7 out]
        n295 = property on="IP" class="Str"() -> ("DisabledEnum"=w421:T3)  [unwired: 2 in, 2 out]
        n296 = case shown="\"Disabled and Grayed Out\"" w421 {
          tunnel: w422 -> [w426 _ _]
          frame "Enabled" {
            n297 = property class="Str"(reference=w426) -> (reference out=w425:refnum<vi>, "Value"=w424:string)  [unwired: 1 in, 1 out]
            n298 = call "字符键盘.vi"("Old String"=w424) -> ("String"=w423:string)  [unwired: 10 in]
            n299 = property class="Str"(reference=w425, "Val(Sgnl)"=w423) -> ()  [unwired: 1 in, 2 out]
          }
          frame "Disabled and Grayed Out" {
            n300 = One Button Dialog(message="关闭连接后才可设置!" ("消息")) -> ()  [unwired: 1 in, 1 out]
          }
          frame "Disabled", Default {
            n301 = One Button Dialog(message="当前操作权限不足,请提升权限!!!" ("消息")) -> ()  [unwired: 1 in, 1 out]
          }
        }
      }
      event "Port": Mouse Down {
        n302 = event-data() -> ("CtlRef"=w430:refnum<vi>)  [unwired: 1 in, 7 out]
        n303 = property on="Port" class="DigNum (严格)"() -> ("DisabledEnum"=w429:T3)  [unwired: 2 in, 2 out]
        n304 = case shown="\"Enabled\"" w429 {
          tunnel: w430 -> [w434 _ _]
          frame "Enabled" {
            n305 = property class="DigNum (严格)"(reference=w434) -> (reference out=w433:refnum<vi>, "Value"=w432:u16)  [unwired: 1 in, 1 out]
            n306 = call "数字键盘.vi"("OldNumber"=w432) -> ("NewNumber"=w431:dbl)  [unwired: 1 in]
            n307 = property class="DigNum (严格)"(reference=w433, "Val(Sgnl)"=w431) -> ()  [unwired: 1 in, 2 out]
          }
          frame "Disabled and Grayed Out" {
            n308 = One Button Dialog(message="关闭连接后才可设置!" ("消息")) -> ()  [unwired: 1 in, 1 out]
          }
          frame "Disabled", Default {
            n309 = One Button Dialog(message="当前操作权限不足,请提升权限!!!" ("消息")) -> ()  [unwired: 1 in, 1 out]
          }
        }
      }
      event "密码锁": Value Change {
        n310 = event-data() -> ("NewVal"=w437:bool)  [unwired: 1 in, 5 out]
        n311 = case shown="假" w437 {
          frame False {
            n312 = global write "多参数全局变量.vi" "权限"(enum16{"一级权限", "二级权限", "三级权限"}."一级权限" ("权限")) -> ()
          }
          frame True {
            n313 = call "数字键盘.vi"("显示样式"=u32 2) -> ("NewNumber"=w442:dbl)  [unwired: 1 in]
            n314 = case shown="23506" w442 {
              tunnel: ["密码错误,即将切换为一级权限!" ("Infoin") "密码正确,即将切换为二级权限!" ("Infoin") "密码正确,即将切换为三级权限!" ("Infoin")] -> w441
              tunnel: [u32 16711680 ("颜色盒") _ _] -> w440
              tunnel: [enum16{"一级权限", "二级权限", "三级权限"}."一级权限" ("权限") enum16{"一级权限", "二级权限", "三级权限"}."二级权限" ("权限") enum16{"一级权限", "二级权限", "三级权限"}."三级权限" ("权限")] -> w439
              frame 0, Default {
              }
              frame 666 {
              }
              frame 23506 {
              }
            }
            n315 = global write "多参数全局变量.vi" "权限"(w439) -> ()
            n316 = call "TimeLmtDialog.vi"("颜色盒"=w440, "Infoin"=w441) -> ()  [unwired: 10 in]
          }
        }
      }
      event "周期设置": Mouse Down {
        n317 = event-data() -> ()  [unwired: 1 in, 6 out]
        n318 = flat-sequence {
          frame #0 {
            n319 = global read "断电保存变量.vi" "定时控制输入"() -> (w452:T6)
            n320 = call "周期设置.vi"("定时控制输入"=w452) -> ("定时控制输出"=w451:T6)  [unwired: 10 in]
            n321 = global write "断电保存变量.vi" "定时控制输入"(w451) -> ()
          }
          frame #1 {
            n322 = call "配置文件保存.vi"() -> ()  [unwired: 12 in]
          }
        }
      }
      event "水样测试": Value Change {
        n323 = event-data() -> ()  [unwired: 1 in, 6 out]
        n324 = vi-ref "水样测试.vi"() -> (w455:refnum<vi>)
        n325 = property class="VI"(reference=w455) -> ("Name"=w459:string, "Exec.State"=w457:T7)  [unwired: 1 in, 2 out]
        n326 = Open VI Reference(type specifier VI Refnum (for type only)=refnum<vi> refnum, vi path=w459, options=128 ("选项")) -> (vi reference=w460:refnum<vi>)  [unwired: 3 in, 1 out]
        n327 = case shown="\"Idle\"" w457 {
          tunnel: [w461 w464] -> w456
          tunnel: w460 -> [w461 w463]
          tunnel: "hd" ("数据标记表") -> [_ w462]
          frame "Bad", Default {
          }
          frame "Idle" {
            n328 = call-by-ref "开始异步调用"(reference=w463, "数据标记表"=w462) -> (reference out=w464:refnum<vi>)  [unwired: 12 in, 1 out]
          }
        }
        n329 = Close Reference(reference=w456) -> ()  [unwired: 1 in, 1 out]
      }
      event "标样核查": Value Change {
        n330 = event-data() -> ()  [unwired: 1 in, 6 out]
        n331 = call "标样核查配置.vi"() -> ("确认输出"=w466:bool, "标样核查配置"=w465:T11)  [unwired: 10 in]
        n332 = case shown="真" w466 {
          tunnel: w465 -> [_ w468]
          frame False {
          }
          frame True {
            n333 = vi-ref "标样核查.vi"() -> (w469:refnum<vi>)
            n334 = property class="VI"(reference=w469) -> ("Name"=w473:string, "Exec.State"=w471:T7)  [unwired: 1 in, 2 out]
            n335 = Open VI Reference(type specifier VI Refnum (for type only)=refnum<vi> refnum, vi path=w473, options=128 ("选项")) -> (vi reference=w474:refnum<vi>)  [unwired: 3 in, 1 out]
            n336 = case shown="\"Idle\"" w471 {
              tunnel: [w475 w478] -> w470
              tunnel: w474 -> [w475 w477]
              tunnel: w468 -> [_ w476]
              frame "Bad", Default {
              }
              frame "Idle" {
                n337 = call-by-ref "开始异步调用"(reference=w477, "标样核查配置"=w476) -> (reference out=w478:refnum<vi>)  [unwired: 12 in, 1 out]
              }
            }
            n338 = Close Reference(reference=w470) -> ()  [unwired: 1 in, 1 out]
          }
        }
      }
      event "停止": Value Change {
        w479 = u16 3 items=["空闲", "水样测试", "标样核查", "停止"] ("主副屏同步启动")
        n339 = event-data() -> ()  [unwired: 1 in, 6 out]
        n340 = Send Notification(notification=TRUE ("通知"), notifier=w481) -> ()  [unwired: 1 in, 2 out]
        n341 = global write "多参数全局变量.vi" "主副屏同步启动"(w479) -> ()
      }
      event "设置": Value Change {
        n342 = event-data() -> ()  [unwired: 1 in, 6 out]
        n343 = property on="窗格" class="Pane"("Origin"=T2 {"Horizontal"=0, "Vertical"=628} ("原点")) -> ()  [unwired: 2 in, 2 out]
      }
      event "pH", "DO", "Turb", "Cond", "Temp", "叶绿素a启用", "藻密度", "VISA资源名称", "连接方式", "IP", "Port", "自动断线重连", "水样测量时间", "ORP启用": Value Change {
        n344 = event-data() -> ()  [unwired: 1 in, 6 out]
        n345 = flat-sequence {
          frame #0 {
            n346 = global write "断电保存变量.vi" "Port"("Port") -> ()
            n347 = global write "断电保存变量.vi" "Temp"("Temp") -> ()
            n348 = global write "断电保存变量.vi" "pH"("pH") -> ()
            n349 = global write "断电保存变量.vi" "orp"("ORP启用") -> ()
            n350 = global write "断电保存变量.vi" "藻密度"("藻密度") -> ()
            n351 = global write "断电保存变量.vi" "IP"("IP") -> ()
            n352 = global write "断电保存变量.vi" "连接方式"("连接方式") -> ()
            n353 = global write "断电保存变量.vi" "DO"("DO") -> ()
            n354 = global write "断电保存变量.vi" "Turb"("Turb") -> ()
            n355 = global write "断电保存变量.vi" "Cond"("Cond") -> ()
            n356 = global write "断电保存变量.vi" "叶绿素a启用"("叶绿素a启用") -> ()
            n357 = global write "断电保存变量.vi" "VISA资源名称"("VISA资源名称") -> ()
            n358 = global write "断电保存变量.vi" "水样测定时间"("水样测量时间") -> ()
            n359 = local read "自动断线重连"() -> (w485:bool)
            n360 = global write "断电保存变量.vi" "自动断线重连"(w485) -> ()
          }
          frame #1 {
            n361 = call "配置文件保存.vi"() -> ()  [unwired: 12 in]
          }
          frame #2 {
          }
        }
      }
      event "打开modbus": Value Change {
        n362 = event-data() -> ()  [unwired: 1 in, 6 out]
        n363 = global read "多参数全局变量.vi" "MB session in"() -> (w503:refnum<class "MB_Master.lvclass">)
        n364 = Flush Queue(queue=w498) -> (queue out=w497:refnum<queue>)  [unwired: 1 in, 2 out]
        n365 = property class="MB_Master"(reference=w503) -> ("Properties:Session Valid"=w502:bool)  [unwired: 1 in, 2 out]
        n366 = Select(t="close" ("元素"), s=w502, f="open" ("元素")) -> (s? t:f=w499:string)
        n367 = Enqueue Element(queue=w497, element=w499) -> ()  [unwired: 2 in, 3 out]
      }
      event "探头校正返回", "设置页返回": Value Change {
        n368 = event-data() -> ()  [unwired: 1 in, 6 out]
        n369 = property on="窗格" class="Pane"("Origin"=T2 {"Horizontal"=0, "Vertical"=0} ("原点")) -> ()  [unwired: 2 in, 2 out]
      }
      event "探头校正", "水温校准": Value Change {
        n370 = event-data() -> ()  [unwired: 1 in, 6 out]
        n371 = property on="窗格" class="Pane"("Origin"=T2 {"Horizontal"=1656, "Vertical"=0} ("原点")) -> ()  [unwired: 2 in, 2 out]
        n372 = vi-ref "水温校准.vi"() -> (w505:refnum<vi>)
        n373 = property class="VI"(reference=w505) -> (reference out=w507:refnum<vi>, "Exec.State"=w506:T7)  [unwired: 1 in, 1 out]
        n374 = case shown="\"Bad\", 默认" w506 {
          tunnel: [w511 w513] -> w509
          tunnel: w507 -> [w511 w512]
          frame "Bad", Default {
          }
          frame "Idle" {
            n375 = invoke class="VI" method="Run VI"(reference=w512, "Wait until done"=FALSE ("结束前等待"), "Auto Dispose Ref"=FALSE ("自动销毁引用")) -> (reference out=w513:refnum<vi>)  [unwired: 2 in, 4 out]
          }
        }
        n376 = invoke on="探头校准子面板" class="SubPnl" method="Remove VI"() -> (error out=w508:errorcluster)  [unwired: 3 in, 2 out]
        n377 = invoke on="探头校准子面板" class="SubPnl" method="Insert VI"(error in=w508, "VI Ref"=w509) -> ()  [unwired: 2 in, 4 out]
      }
      event "pH校准": Value Change {
        n378 = event-data() -> ()  [unwired: 1 in, 6 out]
        n379 = global read "断电保存变量.vi" "探头选择"() -> (w521:T4)
        n380 = Unbundle By Name(w521) -> ("pH探头选择"=w520:u16)
        n381 = case shown="2" w520 {
          tunnel: [w525 w526 w527] -> w519
          frame 0, Default {
            n382 = vi-ref "斯坦道多参数.lvlib:禹山pH校准.vi"() -> (w525:refnum<vi>)
          }
          frame 1 {
            n383 = vi-ref "斯坦道多参数.lvlib:pH电极校准.vi"() -> (w526:refnum<vi>)
          }
          frame 2 {
            n384 = vi-ref "斯坦道多参数.lvlib:纳清pH电极校准.vi"() -> (w527:refnum<vi>)
          }
        }
        n385 = property class="VI"(reference=w519) -> (reference out=w523:refnum<vi>, "Exec.State"=w522:T7)  [unwired: 1 in, 1 out]
        n386 = case shown="\"Bad\", 默认" w522 {
          tunnel: w523 -> [w528 w532]
          tunnel: [w528 w529] -> w517
          frame "Bad", Default {
          }
          frame "Idle" {
            n387 = invoke class="VI" method="Run VI"(reference=w532, "Wait until done"=FALSE ("结束前等待"), "Auto Dispose Ref"=FALSE ("自动销毁引用")) -> (reference out=w529:refnum<vi>)  [unwired: 2 in, 4 out]
          }
        }
        n388 = global read "多参数全局变量.vi" "校准VI引用句柄"() -> (w518:T10)
        n389 = invoke on="探头校准子面板" class="SubPnl" method="Remove VI"() -> (error out=w524:errorcluster)  [unwired: 3 in, 2 out]
        n390 = invoke on="探头校准子面板" class="SubPnl" method="Insert VI"(error in=w524, "VI Ref"=w517) -> ()  [unwired: 2 in, 4 out]
        n391 = Bundle By Name(cluster=w518, "pH校准VI引用句柄"=w517) -> (w516:T10)
        n392 = global write "多参数全局变量.vi" "校准VI引用句柄"(w516) -> ()
      }
      event "电导率校准": Value Change {
        n393 = event-data() -> ()  [unwired: 1 in, 6 out]
        n394 = global read "断电保存变量.vi" "探头选择"() -> (w538:T4)
        n395 = Unbundle By Name(w538) -> ("电导率探头选择"=w537:u16)
        n396 = case shown="2" w537 {
          tunnel: [w542 w543 w544] -> w536
          frame 0, Default {
            n397 = vi-ref "斯坦道多参数.lvlib:禹山电导率校准.vi"() -> (w542:refnum<vi>)
          }
          frame 1 {
            n398 = vi-ref "斯坦道多参数.lvlib:电导率电极校准.vi"() -> (w543:refnum<vi>)
          }
          frame 2 {
            n399 = vi-ref "斯坦道多参数.lvlib:纳清电导率电极校准.vi"() -> (w544:refnum<vi>)
          }
        }
        n400 = property class="VI"(reference=w536) -> (reference out=w540:refnum<vi>, "Exec.State"=w539:T7)  [unwired: 1 in, 1 out]
        n401 = case shown="\"Bad\", 默认" w539 {
          tunnel: [w545 w547] -> w533
          tunnel: w540 -> [w545 w546]
          frame "Bad", Default {
          }
          frame "Idle" {
            n402 = invoke class="VI" method="Run VI"(reference=w546, "Wait until done"=FALSE ("结束前等待"), "Auto Dispose Ref"=FALSE ("自动销毁引用")) -> (reference out=w547:refnum<vi>)  [unwired: 2 in, 4 out]
          }
        }
        n403 = global read "多参数全局变量.vi" "校准VI引用句柄"() -> (w535:T10)
        n404 = invoke on="探头校准子面板" class="SubPnl" method="Remove VI"() -> (error out=w541:errorcluster)  [unwired: 3 in, 2 out]
        n405 = Bundle By Name(cluster=w535, "COND校准VI引用句柄"=w533) -> (w534:T10)
        n406 = invoke on="探头校准子面板" class="SubPnl" method="Insert VI"(error in=w541, "VI Ref"=w533) -> ()  [unwired: 2 in, 4 out]
        n407 = global write "多参数全局变量.vi" "校准VI引用句柄"(w534) -> ()
      }
      event "溶解氧校准": Value Change {
        n408 = event-data() -> ()  [unwired: 1 in, 6 out]
        n409 = global read "断电保存变量.vi" "探头选择"() -> (w555:T4)
        n410 = Unbundle By Name(w555) -> ("DO探头选择"=w554:u16)
        n411 = case shown="2" w554 {
          tunnel: [w559 w560 w561] -> w553
          frame 0, Default {
            n412 = vi-ref "斯坦道多参数.lvlib:禹山溶解氧校准.vi"() -> (w559:refnum<vi>)
          }
          frame 1 {
            n413 = vi-ref "斯坦道多参数.lvlib:溶解氧电极校准.vi"() -> (w560:refnum<vi>)
          }
          frame 2 {
            n414 = vi-ref "斯坦道多参数.lvlib:纳清DO电极校准.vi"() -> (w561:refnum<vi>)
          }
        }
        n415 = property class="VI"(reference=w553) -> (reference out=w557:refnum<vi>, "Exec.State"=w556:T7)  [unwired: 1 in, 1 out]
        n416 = case shown="\"Bad\", 默认" w556 {
          tunnel: [w562 w564] -> w550
          tunnel: w557 -> [w562 w563]
          frame "Bad", Default {
          }
          frame "Idle" {
            n417 = invoke class="VI" method="Run VI"(reference=w563, "Wait until done"=FALSE ("结束前等待"), "Auto Dispose Ref"=FALSE ("自动销毁引用")) -> (reference out=w564:refnum<vi>)  [unwired: 2 in, 4 out]
          }
        }
        n418 = global read "多参数全局变量.vi" "校准VI引用句柄"() -> (w552:T10)
        n419 = invoke on="探头校准子面板" class="SubPnl" method="Remove VI"() -> (error out=w558:errorcluster)  [unwired: 3 in, 2 out]
        n420 = invoke on="探头校准子面板" class="SubPnl" method="Insert VI"(error in=w558, "VI Ref"=w550) -> ()  [unwired: 2 in, 4 out]
        n421 = Bundle By Name(cluster=w552, "DO校准VI引用句柄"=w550) -> (w551:T10)
        n422 = global write "多参数全局变量.vi" "校准VI引用句柄"(w551) -> ()
      }
      event "浊度校准": Value Change {
        n423 = event-data() -> ()  [unwired: 1 in, 6 out]
        n424 = global read "断电保存变量.vi" "探头选择"() -> (w572:T4)
        n425 = Unbundle By Name(w572) -> ("浊度探头选择"=w571:u16)
        n426 = case shown="2" w571 {
          tunnel: [w576 w577 w578] -> w570
          frame 0, Default {
            n427 = vi-ref "斯坦道多参数.lvlib:禹山浊度校准.vi"() -> (w576:refnum<vi>)
          }
          frame 1 {
            n428 = vi-ref "斯坦道多参数.lvlib:浊度电极校准.vi"() -> (w577:refnum<vi>)
          }
          frame 2 {
            n429 = vi-ref "斯坦道多参数.lvlib:纳清浊度电极校准.vi"() -> (w578:refnum<vi>)
          }
        }
        n430 = property class="VI"(reference=w570) -> (reference out=w574:refnum<vi>, "Exec.State"=w573:T7)  [unwired: 1 in, 1 out]
        n431 = case shown="\"Bad\", 默认" w573 {
          tunnel: [w579 w581] -> w567
          tunnel: w574 -> [w579 w580]
          frame "Bad", Default {
          }
          frame "Idle" {
            n432 = invoke class="VI" method="Run VI"(reference=w580, "Wait until done"=FALSE ("结束前等待"), "Auto Dispose Ref"=FALSE ("自动销毁引用")) -> (reference out=w581:refnum<vi>)  [unwired: 2 in, 4 out]
          }
        }
        n433 = global read "多参数全局变量.vi" "校准VI引用句柄"() -> (w569:T10)
        n434 = invoke on="探头校准子面板" class="SubPnl" method="Remove VI"() -> (error out=w575:errorcluster)  [unwired: 3 in, 2 out]
        n435 = invoke on="探头校准子面板" class="SubPnl" method="Insert VI"(error in=w575, "VI Ref"=w567) -> ()  [unwired: 2 in, 4 out]
        n436 = Bundle By Name(cluster=w569, "TURB校准VI引用句柄"=w567) -> (w568:T10)
        n437 = global write "多参数全局变量.vi" "校准VI引用句柄"(w568) -> ()
      }
      event "叶绿素a校准": Value Change {
        n438 = event-data() -> ()  [unwired: 1 in, 6 out]
        n439 = global read "断电保存变量.vi" "探头选择"() -> (w588:T4)
        n440 = Unbundle By Name(w588) -> ("叶绿素a探头选择"=w587:u16)
        n441 = case shown="2" w587 {
          tunnel: [w593 _ w594] -> w589
          frame 0, Default {
            n442 = vi-ref "禹山叶绿素a校准.vi"() -> (w593:refnum<vi>)
          }
          frame 1 {
          }
          frame 2 {
            n443 = vi-ref "斯坦道多参数.lvlib:纳清叶绿素a电极校准.vi"() -> (w594:refnum<vi>)
          }
        }
        n444 = property class="VI"(reference=w589) -> (reference out=w591:refnum<vi>, "Exec.State"=w590:T7)  [unwired: 1 in, 1 out]
        n445 = case shown="\"Bad\", 默认" w590 {
          tunnel: [w595 w597] -> w584
          tunnel: w591 -> [w595 w596]
          frame "Bad", Default {
          }
          frame "Idle" {
            n446 = invoke class="VI" method="Run VI"(reference=w596, "Wait until done"=FALSE ("结束前等待"), "Auto Dispose Ref"=FALSE ("自动销毁引用")) -> (reference out=w597:refnum<vi>)  [unwired: 2 in, 4 out]
          }
        }
        n447 = global read "多参数全局变量.vi" "校准VI引用句柄"() -> (w586:T10)
        n448 = invoke on="探头校准子面板" class="SubPnl" method="Remove VI"() -> (error out=w592:errorcluster)  [unwired: 3 in, 2 out]
        n449 = invoke on="探头校准子面板" class="SubPnl" method="Insert VI"(error in=w592, "VI Ref"=w584) -> ()  [unwired: 2 in, 4 out]
        n450 = Bundle By Name(cluster=w586, "CHLA校准VI引用句柄"=w584) -> (w585:T10)
        n451 = global write "多参数全局变量.vi" "校准VI引用句柄"(w585) -> ()
      }
      event "藻密度校准": Value Change {
        n452 = event-data() -> ()  [unwired: 1 in, 6 out]
        n453 = global read "断电保存变量.vi" "探头选择"() -> (w604:T4)
        n454 = Unbundle By Name(w604) -> ("蓝绿藻探头选择"=w603:u16)
        n455 = case shown="2" w603 {
          tunnel: [_ w609] -> w605
          frame 0, Default {
          }
          frame 2 {
            n456 = vi-ref "斯坦道多参数.lvlib:纳清蓝绿藻电极校准.vi"() -> (w609:refnum<vi>)
          }
        }
        n457 = property class="VI"(reference=w605) -> (reference out=w607:refnum<vi>, "Exec.State"=w606:T7)  [unwired: 1 in, 1 out]
        n458 = case shown="\"Bad\", 默认" w606 {
          tunnel: [w610 w612] -> w600
          tunnel: w607 -> [w610 w611]
          frame "Bad", Default {
          }
          frame "Idle" {
            n459 = invoke class="VI" method="Run VI"(reference=w611, "Wait until done"=FALSE ("结束前等待"), "Auto Dispose Ref"=FALSE ("自动销毁引用")) -> (reference out=w612:refnum<vi>)  [unwired: 2 in, 4 out]
          }
        }
        n460 = global read "多参数全局变量.vi" "校准VI引用句柄"() -> (w602:T10)
        n461 = invoke on="探头校准子面板" class="SubPnl" method="Remove VI"() -> (error out=w608:errorcluster)  [unwired: 3 in, 2 out]
        n462 = invoke on="探头校准子面板" class="SubPnl" method="Insert VI"(error in=w608, "VI Ref"=w600) -> ()  [unwired: 2 in, 4 out]
        n463 = Bundle By Name(cluster=w602, "BGA校准VI引用句柄"=w600) -> (w601:T10)
        n464 = global write "多参数全局变量.vi" "校准VI引用句柄"(w601) -> ()
      }
      event "ORP校准": Value Change {
        n465 = event-data() -> ()  [unwired: 1 in, 6 out]
        n466 = global read "断电保存变量.vi" "探头选择"() -> (w619:T4)
        n467 = Unbundle By Name(w619) -> ("orp探头选择"=w618:u16)
        n468 = case shown="1" w618 {
          tunnel: [_ w624] -> w620
          frame 0, Default {
          }
          frame 1 {
            n469 = vi-ref "斯坦道多参数.lvlib:ORP电极校准.vi"() -> (w624:refnum<vi>)
          }
        }
        n470 = property class="VI"(reference=w620) -> (reference out=w622:refnum<vi>, "Exec.State"=w621:T7)  [unwired: 1 in, 1 out]
        n471 = case shown="\"Bad\", 默认" w621 {
          tunnel: [w625 w627] -> w615
          tunnel: w622 -> [w625 w626]
          frame "Bad", Default {
          }
          frame "Idle" {
            n472 = invoke class="VI" method="Run VI"(reference=w626, "Wait until done"=FALSE ("结束前等待"), "Auto Dispose Ref"=FALSE ("自动销毁引用")) -> (reference out=w627:refnum<vi>)  [unwired: 2 in, 4 out]
          }
        }
        n473 = global read "多参数全局变量.vi" "校准VI引用句柄"() -> (w617:T10)
        n474 = invoke on="探头校准子面板" class="SubPnl" method="Remove VI"() -> (error out=w623:errorcluster)  [unwired: 3 in, 2 out]
        n475 = Bundle By Name(cluster=w617, "ORP校准VI引用句柄"=w615) -> (w616:T10)
        n476 = invoke on="探头校准子面板" class="SubPnl" method="Insert VI"(error in=w623, "VI Ref"=w615) -> ()  [unwired: 2 in, 4 out]
        n477 = global write "多参数全局变量.vi" "校准VI引用句柄"(w616) -> ()
      }
    }
  }
  n478 = property on="编号" class="Str"("Visible"=w1) -> ()  [unwired: 2 in, 2 out]
  n479 = while {
    tunnel: [w637] -> _
    shift-right: [w635] -> _
    shift-left: _ -> [w634]
    tunnel: w4 -> [w631]
    stop <- FALSE stop-if-true
    n480 = Wait (ms)(milliseconds to wait=u32 1000 ("等待时间（毫秒）")) -> ()  [unwired: 1 out]
    n481 = global read "多参数全局变量.vi" "配置文件 path"() -> (w630:path)
    n482 = Get File Size(file=w630, error in=w631) -> (size (in bytes)=w635:i64, 0:w632:errorcluster)  [unwired: 1 out]
    n483 = Not Equal?(x=w635, y=w634) -> (x != y?=w633:bool)
    n484 = case shown="真" w633 {
      tunnel: [w639 w643] -> w637
      tunnel: w630 -> [_ w642]
      tunnel: w632 -> [w639 w641]
      frame False {
      }
      frame True {
        # "文件发生改变进行更新"
        n485 = call <vilib>:"Open Config Data.vi"("error in (no error)"=w641, "configuration file path"=w642) -> ("error out"=w647:errorcluster, "refnum"=w646:T9)  [unwired: 7 in, 1 out]
        n486 = vi-ref "断电保存变量.vi"() -> (w640:refnum<vi>)
        n487 = call <userlib>:"Read Panel from INI__ogtk.vi"("error in (no error)"=w647, "VI ref"=w640, "refnum"=w646) -> ("error out"=w645:errorcluster, "refnum out"=w644:T9)  [unwired: 7 in]
        n488 = call <vilib>:"Close Config Data.vi"("error in (no error)"=w645, "refnum"=w644) -> ("error out"=w643:errorcluster)  [unwired: 8 in, 1 out]
      }
    }
  }
  n489 = while {
    tunnel: w36 -> [w649]
    tunnel: w4 -> [_]
    stop <- FALSE stop-if-true
    n490 = Dequeue Element(queue=w649) -> (element=w648:string)  [unwired: 2 in, 3 out]
    n491 = case shown="\"open\"" w648 {
      tunnel: [_ w651 w661] -> _
      frame "假", Default {
      }
      frame "open" {
        n492 = global read "多参数全局变量.vi" "MB session in"() -> (w656:refnum<class "MB_Master.lvclass">)
        n493 = global read "断电保存变量.vi" "VISA资源名称"() -> (w658:refnum<visa-resource-name>)
        n494 = global read "断电保存变量.vi" "连接方式"() -> (w654:u16)
        n495 = call "close MB.vi"("MB session in"=w656) -> ("error out"=w659:errorcluster)  [unwired: 10 in]
        n496 = global read "断电保存变量.vi" "Port"() -> (w652:u16)
        n497 = global read "断电保存变量.vi" "IP"() -> (w653:string)
        n498 = call "open MB.vi"("Port (502)"=w652, "IP Address"=w653, "MODE"=w654, "error in (no error)"=w659, "Serial Config"=T12 {"baud rate (bps)"=9600, "stop bits"=10, "parity"=0, "flow control"=0, "timeout"=1000, "retries"=1}, "VISA资源名称"=w658) -> ("error out"=w651:errorcluster, "MB session out"=w655:refnum<class "MB_Master.lvclass">)  [unwired: 4 in]
        n499 = global write "多参数全局变量.vi" "MB session in"(w655) -> ()
      }
      frame "close" {
        n500 = global read "多参数全局变量.vi" "MB session in"() -> (w660:refnum<class "MB_Master.lvclass">)
        n501 = call "close MB.vi"("MB session in"=w660) -> ("error out"=w661:errorcluster)  [unwired: 10 in]
      }
    }
  }
  n502 = while {
    tunnel: w36 -> [w663]
    stop <- FALSE stop-if-true
    # "断线重连"
    n503 = global read "断电保存变量.vi" "连接方式"() -> (w664:u16)
    n504 = Wait (ms)(milliseconds to wait=u32 10000 ("等待时间（毫秒）")) -> ()  [unwired: 1 out]
    n505 = case shown="1" w664 {
      tunnel: w663 -> [_ w667]
      frame 0, Default {
      }
      frame 1 {
        n506 = case shown="真" "自动断线重连" {
          tunnel: w667 -> [_ w670]
          frame False {
          }
          frame True {
            n507 = global read "多参数全局变量.vi" "MB session in"() -> (w669:refnum<class "MB_Master.lvclass">)
            n508 = property class="MB_Master"(reference=w669) -> ("Properties:Session Valid"=w668:bool)  [unwired: 1 in, 2 out]
            n509 = case shown="假" w668 {
              tunnel: w670 -> [w671 _]
              frame False {
                n510 = Flush Queue(queue=w671) -> (queue out=w673:refnum<queue>)  [unwired: 1 in, 2 out]
                n511 = Enqueue Element(queue=w673, element="open" ("元素")) -> ()  [unwired: 2 in, 3 out]
              }
              frame True {
              }
            }
          }
        }
      }
    }
  }
